vi "main.vi"() -> ()   [LabVIEW 2018]
uses:
  <vilib>/Platform/TimedLoop/XDataNode/timing_clust.ctl
  <vilib>/Platform/TimedLoop/XDataNode/nitl_modes.ctl
  <vilib>/Platform/TimedLoop/XDataNode/wakeup.ctl
  <vilib>/rvi/Emulation/niFpgaGetClockAttributes.vi
  <vilib>/rvi/Emulation/niFpgaSctlEmulationGetInTimedLoop.vi
  <vilib>/rvi/Emulation/niFpgaEmulationReportErrorSimple.vi
  <vilib>/rvi/Emulation/niFpgaProcessEmulError.vi
  <vilib>/rvi/Emulation/niFpgaCriticalErrorInLSC.vi
  <vilib>/Platform/TimedLoop/XDataNode/XDataNode.xnode
  <vilib>/Platform/TimedLoop/XDataNode/XDNodeRunTimeDep.lvlib
panel:
  out "fxp_T_extra2":i32
  out "fxp_T_extra1":i32
  out "fxp_T_pneum":i32
  out "fxp_T_pod":i32
  out "fxp_T_avb_r":i32
  out "fxp_T_avb_p2":i32
  out "fxp_T_avb_p1":i32
  out "fxp_T_piston7":i32
  out "fxp_T_piston6":i32
  out "fxp_T_piston5":i32
  out "fxp_T_piston4":i32
  out "fxp_T_piston3":i32
  out "fxp_T_piston2":i32
  out "fxp_T_piston1":i32
  out "fxp_T_piston0":i32
  out "fuse_avb_p2":bool
  out "fuse_avb_p1":bool
  out "frg_run_state":bool=TRUE
  in  "frg_run":bool=TRUE
  out "cur_thresh_index":u8
  out "cur_thresh_persistence":u32
  out "cur_thresh_ratio":u32
  out "fxp_cur_thresh_max":i32
  out "fxp_cur_thresh_min":i32
  out "fxp_fusion_distance":i32
  in  "fxp_mc_linear_v":i32
  out "fxp_mc_distance":i32
  out "fxp_imu_distance":i32
  in  "fxp_imu_acc":i32
  in  "reset_tape_status":bool
  out "light_sensor_status":u8
  out "enable_checks_state":bool
  in  "enable_checks":bool
  out "fxp_brake_distance":i32
  out "fxp_tape_distance":i32
  out "fxp_brake_force":i32
  out "fxp_P_lp2":i32
  out "fxp_P_lp1":i32
  out "fxp_P_hp2":i32
  out "fxp_P_hp1":i32
  out "fxp_T_cRIO":i32
  out "fxp_tape_velocity":i32
  out "light_R_count":u8
  out "light_L_count":u8
  out "light_BR_count":u8
  out "light_BL_count":u8
  out "light_FL_count":u8
  in  "hvr_4":bool
  in  "hvr_3":bool
  in  "hvr_2":bool
  in  "hvr_1":bool
  in  "avb_shutoff_res":bool
  in  "avb_shutoff_prim_2":bool
  in  "avb_shutoff_prim_1":bool
  in  "iso_led_2":bool
  in  "iso_led_1":bool
  out "avb_shutoff_r_state":bool
  out "avb_shutoff_p2_state":bool
  out "avb_shutoff_p1_state":bool
  out "iso_led_2_state":bool
  out "iso_led_1_state":bool
  out "HVR_4_state":bool
  out "HVR_3_state":bool
  out "HVR_2_state":bool
  out "HVR_1_state":bool
  out "drain_valve_state":bool
  out "brake_state":bool
  out "fxp_voltage_r":i32
  out "fxp_voltage_p2":i32
  out "fxp_voltage_p1":i32
  out "fault_long_3":u64
  out "fault_long_2":u64
  out "soft_fault":u64
  out "hard_fault":u64
  in  "value":fxp<+/-,32,16>
  in  "thresh_read_index":u8
  in  "thresh_reset":bool
  in  "thresh_reset_index":u8
  in  "thresh_latch_new":bool
  in  "thresh_f_ratio":u32
  in  "thresh_persistence":u32
  in  "fxp_thresh_new_max":i32
  in  "fxp_thresh_new_min":i32
  in  "thresh_write_index":u8
  in  "stop":bool
  out "fxp_current_r":i32
  out "fxp_current_p2":i32
  out "fxp_current_p1":i32
  in  "actuate_drain":bool
  in  "actuate_brakes":bool
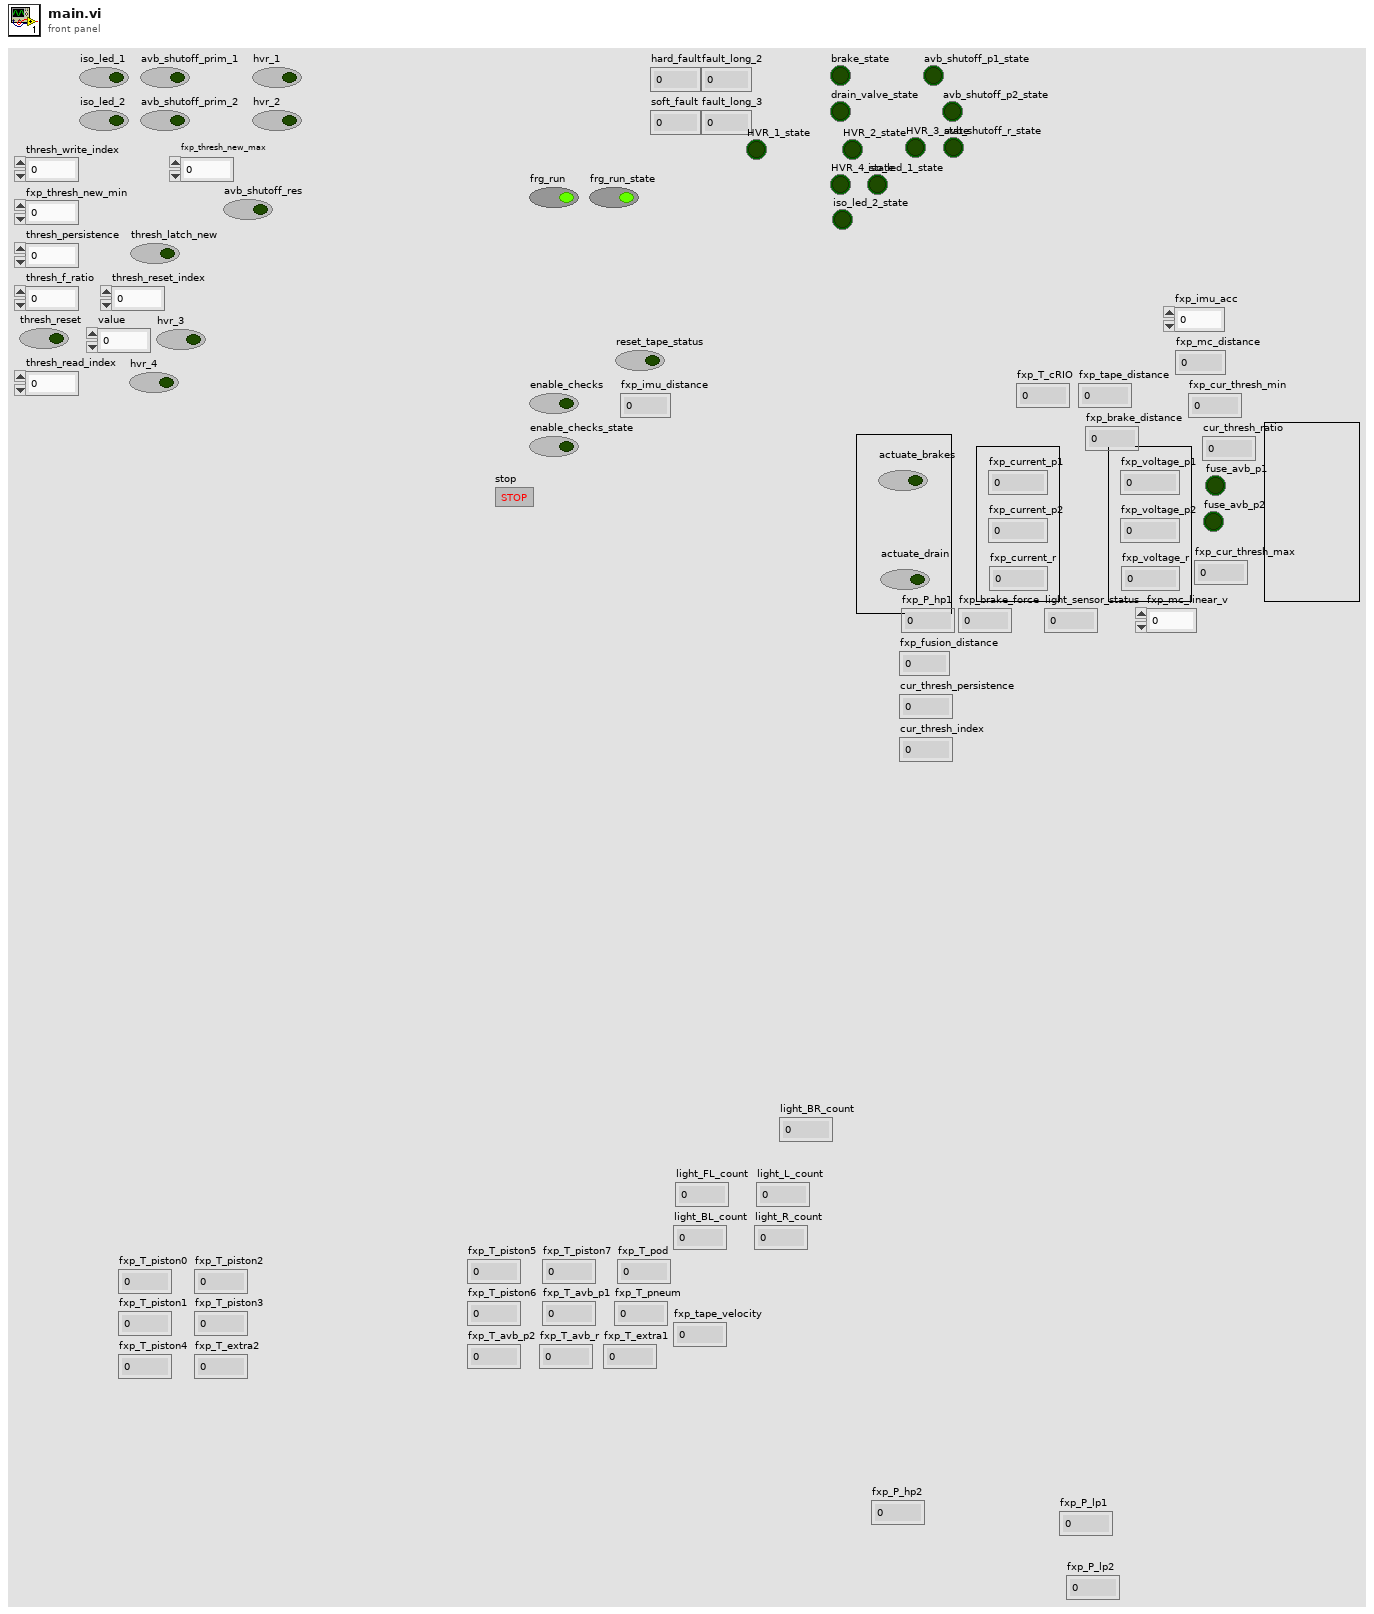
[diagram p1: front panel]
types:
  T1 = typedef "XDNodeRunTimeDep.lvlib/timing_clust.ctl" = cluster{"Expected End [f-1]":u64, "Actual End [f-1]":u64, "Finished Late? [f-1]":bool, "Expected End [i-1]":u64, "Actual End [i-1]":u64, "Finished Late? [i-1]":bool, "Expected Start [i]":u64, "Actual Start [i]":u64, "Expected Start [f]":u64, "Actual Start [f]":u64, "Source Name":string, "Structure Name":string, "Period":i64, "Deadline":i64, "Offset":i64, "Start":i64, "Priority":i32, "Timeout":i32, "Mode":T2, "Wakeup Reason":T3, "Error":errorcluster, "Source Type":string, "Secondary Source Type":string, "Global End Time":u64, "Global Start Time":u64, "Frame Duration":u64, "Iteration Duration":u64, "Assigned CPU":i32, "I/O Scan Engine Mode":u32}
  T2 = typedef "XDNodeRunTimeDep.lvlib/nitl_modes.ctl" = enum32{"No Change", "Process missed periods, maintain original phase", "Discard missed periods, maintain original phase", "Process missed periods, ignore original phase", "Discard missed periods, ignore original phase"}
  T3 = typedef "XDNodeRunTimeDep.lvlib/wakeup.ctl" = enum32{"Normal", "Aborted", "Asynchronous wakeup", "Timing source error", "Timed loop error", "Timeout"}
  T4 = typedef "validated_analog.ctl" = cluster{"valid":bool, "analog":fxp<+/-,24,5>}
  T5 = typedef "validated_bool.ctl" = cluster{"valid":bool, "bool":bool}
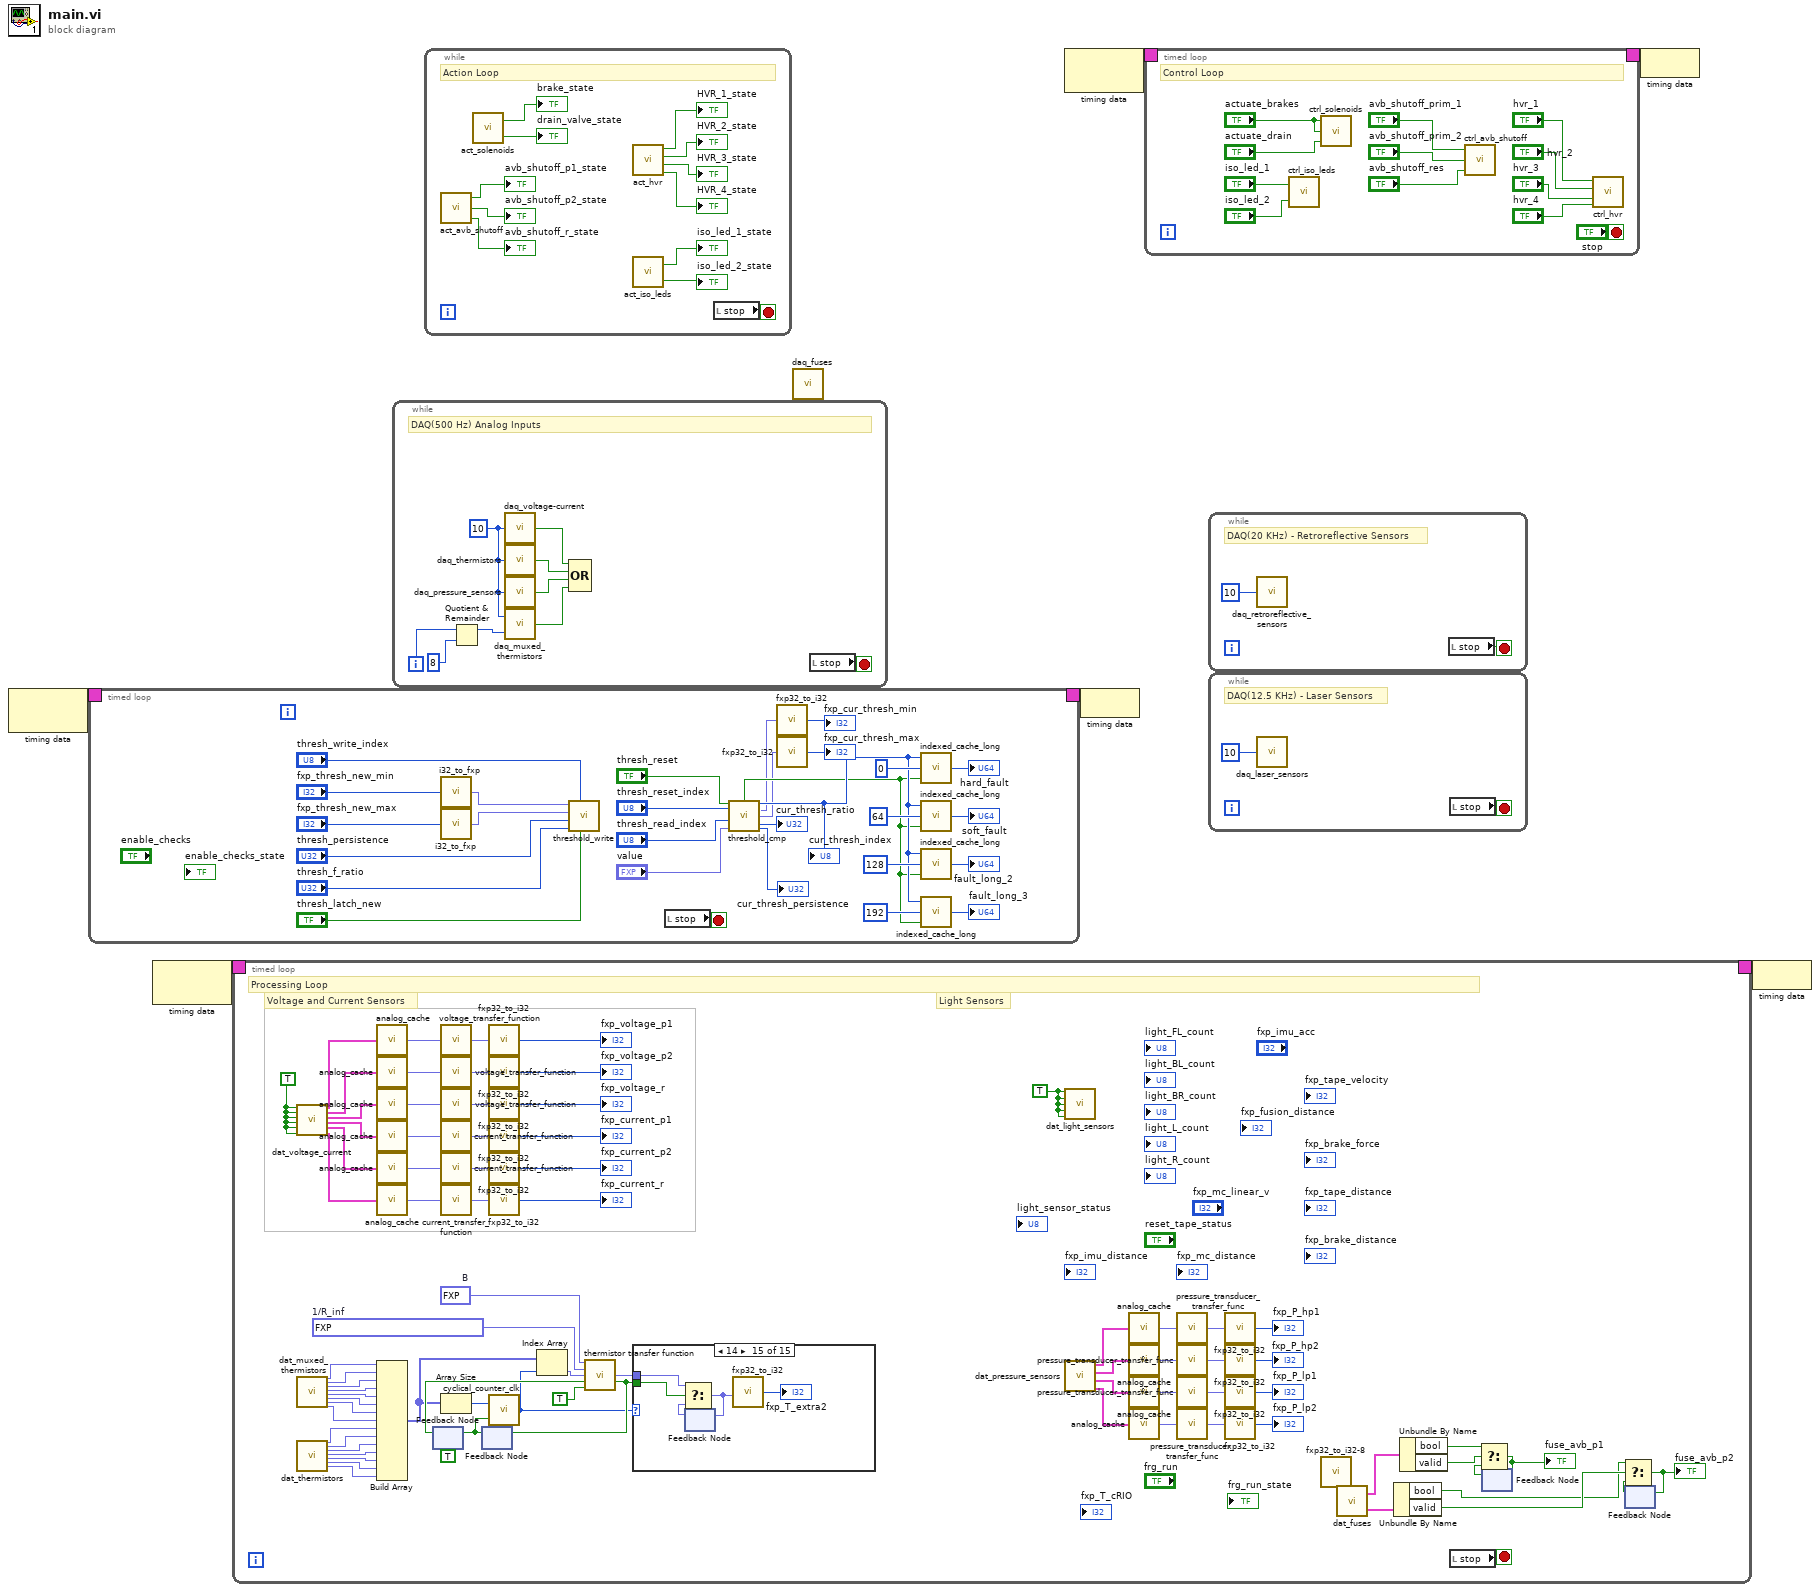
[diagram p0: block diagram]
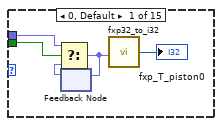
[diagram p2: hidden frame]
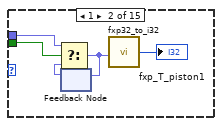
[diagram p3: hidden frame]
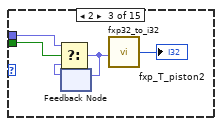
[diagram p4: hidden frame]
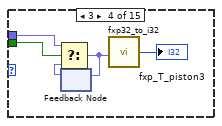
[diagram p5: hidden frame]
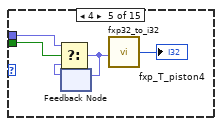
[diagram p6: hidden frame]
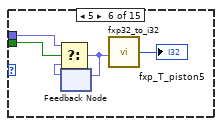
[diagram p7: hidden frame]
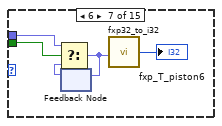
[diagram p8: hidden frame]
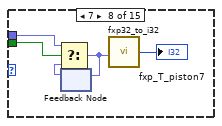
[diagram p9: hidden frame]
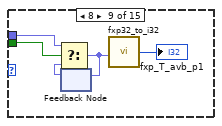
[diagram p10: hidden frame]
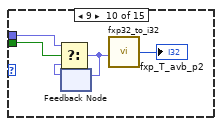
[diagram p11: hidden frame]
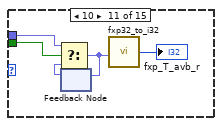
[diagram p12: hidden frame]
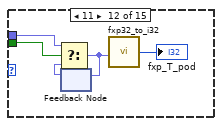
[diagram p13: hidden frame]
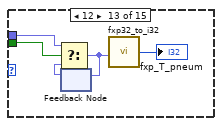
[diagram p14: hidden frame]
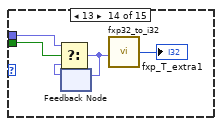
[diagram p15: hidden frame]
diagram:
  n1 = node-c288() -> (w2:T1)  [unwired: 1 in]
  n2 = timed-loop {
    timing: w2 -> [_]
    timing-out: [_] -> w1
    stop <- w35 stop-if-true
    n3 = call "i32_to_fxp.vi"("32bit integer"="fxp_thresh_new_min") -> ("fxp32_16"=w14:fxp<+/-,32,16>)
    n4 = call "i32_to_fxp.vi"("32bit integer"="fxp_thresh_new_max") -> ("fxp32_16"=w13:fxp<+/-,32,16>)
    n5 = call "threshold_write.vi"("thresh_latch"="thresh_latch_new", "thresh_index"="thresh_write_index", "thresh_f_ratio"="thresh_f_ratio", "thresh_persistence"="thresh_persistence", "thresh_new_max"=w13, "thresh_new_min"=w14) -> ()  [unwired: 4 in]
    n6 = local read "stop"() -> (w35:bool)
    n7 = call "threshold_cmp.vi"("thresh_reset"="thresh_reset", "thresh_reset_index"="thresh_reset_index", "index"="thresh_read_index", "value"="value") -> ("thresh_fault"=w21:bool, "current_index"=w22:u8, "current_minimum"=w10:fxp<+/-,32,16>, "current_maximum"=w9:fxp<+/-,32,16>, "current_ratio"=→"cur_thresh_ratio":u32, "current_persistence"=→"cur_thresh_persistence":u32)  [unwired: 6 in]
    "cur_thresh_index" <- w22
    n8 = call "fxp32_to_i32.vi"("fxp32_16"=w10) -> ("32bit integer"=→"fxp_cur_thresh_min":i32)
    n9 = call "fxp32_to_i32.vi"("fxp32_16"=w9) -> ("32bit integer"=→"fxp_cur_thresh_max":i32)
    n10 = call "indexed_cache_long.vi"("bool"=w21, "start index"=u8 0, "index"=w22) -> ("long"=→"hard_fault":u64)  [unwired: 2 in]
    n11 = call "indexed_cache_long.vi"("bool"=w21, "start index"=u8 64, "index"=w22) -> ("long"=→"soft_fault":u64)  [unwired: 2 in]
    n12 = call "indexed_cache_long.vi"("bool"=w21, "start index"=u8 128, "index"=w22) -> ("long"=→"fault_long_2":u64)  [unwired: 2 in]
    n13 = call "indexed_cache_long.vi"("bool"=w21, "start index"=u8 192, "index"=w22) -> ("long"=→"fault_long_3":u64)  [unwired: 2 in]
  }
  n14 = node-c288() -> (w4:T1)  [unwired: 1 in]
  n15 = timed-loop {
    timing: w4 -> [_]
    timing-out: [_] -> w3
    stop <- w111 stop-if-true
    w47 = fxp<+,32,7> 10.047783523797989  # 1/R_inf
    w48 = fxp<+/-,32,16> 3434.0  # B
    w91 = TRUE ("FL-Ready for Output")
    w92 = TRUE
    # "Voltage and Current Sensors"
    # "Light Sensors"
    # "Processing Loop"
    n16 = call "dat_voltage_current.vi"("P1-V Ready for Output"=w92, "P2-V Ready for Output"=w92, "R-V Ready for Output"=w92, "P1-C Ready for Output"=w92, "P2-C Ready for Output"=w92, "R-C Ready for Output"=w92) -> ("P1-V"=w98:T4, "P2-V"=w93:T4, "R-V"=w94:T4, "P1-C"=w95:T4, "P2-C"=w96:T4, "R-C"=w97:T4)  [unwired: 8 in]
    n17 = call "dat_muxed_thermistors.vi"() -> ("v_piston_0"=w64:fxp<+/-,24,5>, "v_piston_1"=w63:fxp<+/-,24,5>, "v_piston_2"=w62:fxp<+/-,24,5>, "v_piston_3"=w61:fxp<+/-,24,5>, "v_piston_4"=w60:fxp<+/-,24,5>, "v_piston_5"=w59:fxp<+/-,24,5>, "v_piston_6"=w58:fxp<+/-,24,5>, "v_piston_7"=w57:fxp<+/-,24,5>)  [unwired: 20 in]
    n18 = call "dat_thermistors.vi"() -> ("v_pb_1_t"=w56:fxp<+/-,24,5>, "v_pb_2_t"=w55:fxp<+/-,24,5>, "v_rb_t"=w54:fxp<+/-,24,5>, "v_pod_t"=w53:fxp<+/-,24,5>, "v_pneum_tank_t"=w52:fxp<+/-,24,5>, "v_extra_1_t"=w51:fxp<+/-,24,5>, "v_extra_2_t"=w50:fxp<+/-,24,5>)  [unwired: 20 in, 1 out]
    n19 = call "analog_cache.vi"("Cluster"=w98) -> ("$_val"=w104:fxp<+/-,24,5>)
    n20 = call "analog_cache.vi"("Cluster"=w93) -> ("$_val"=w103:fxp<+/-,24,5>)
    n21 = call "analog_cache.vi"("Cluster"=w94) -> ("$_val"=w102:fxp<+/-,24,5>)
    n22 = call "analog_cache.vi"("Cluster"=w95) -> ("$_val"=w101:fxp<+/-,24,5>)
    n23 = call "analog_cache.vi"("Cluster"=w96) -> ("$_val"=w100:fxp<+/-,24,5>)
    n24 = call "analog_cache.vi"("Cluster"=w97) -> ("$_val"=w99:fxp<+/-,24,5>)
    n25 = Build Array(w64, w63, w62, w61, w60, w59, w58, w57, w56, w55, w54, w53, w52, w51, w50) -> (w38:fxp<+/-,24,5>[])
    n26 = feedback #1(TRUE ("ready for input")) -> (w42:bool)
    n27 = call "voltage_transfer_function.vi"("V_in"=w104) -> ("V"=w107:fxp<+/-,32,16>)
    n28 = call "voltage_transfer_function.vi"("V_in"=w103) -> ("V"=w106:fxp<+/-,32,16>)
    n29 = call "voltage_transfer_function.vi"("V_in"=w102) -> ("V"=w105:fxp<+/-,32,16>)
    n30 = call "current_transfer_function.vi"("V_in"=w101) -> ("I"=w114:fxp<+/-,32,16>)
    n31 = call "current_transfer_function.vi"("V_in"=w100) -> ("I"=w113:fxp<+/-,32,16>)
    n32 = call "current_transfer_function.vi"("V_in"=w99) -> ("I"=w112:fxp<+/-,32,16>)
    n33 = Array Size(array=w38) -> (size(s)=w45:i32)
    n34 = feedback #2() -> (w40:bool)  [unwired: 1 in]
    n35 = feedback-in #1(w40) -> ()
    n36 = call "fxp32_to_i32.vi"("fxp32_16"=w107) -> ("32bit integer"=→"fxp_voltage_p1":i32)
    n37 = call "fxp32_to_i32.vi"("fxp32_16"=w106) -> ("32bit integer"=→"fxp_voltage_p2":i32)
    n38 = call "fxp32_to_i32.vi"("fxp32_16"=w105) -> ("32bit integer"=→"fxp_voltage_r":i32)
    n39 = call "fxp32_to_i32.vi"("fxp32_16"=w114) -> ("32bit integer"=→"fxp_current_p1":i32)
    n40 = call "fxp32_to_i32.vi"("fxp32_16"=w113) -> ("32bit integer"=→"fxp_current_p2":i32)
    n41 = call "fxp32_to_i32.vi"("fxp32_16"=w112) -> ("32bit integer"=→"fxp_current_r":i32)
    n42 = call "cyclical_counter_clk.vi"("clk"=w40, "Mod"=w45) -> ("Count"=w39:u16)
    n43 = Index Array(array=w38, index=w39) -> (element=w49:fxp<+/-,24,5>)
    n44 = call "thermistor transfer function.vi"("B"=w48, "1/R_inf"=w47, "V"=w49, "input valid"=w42, "ready for output (T)"=TRUE) -> ("Temperature"=w46:fxp<+/-,32,16>, "output valid"=w41:bool)  [unwired: 8 in, 1 out]
    n45 = feedback-in #2(w41) -> ()
    n46 = case shown="14" w39 {
      tunnel: w41 -> [w119 w124 w129 w134 w139 w144 w149 w154 w159 w164 w169 w174 w179 w184 w189]
      tunnel: w46 -> [w122 w127 w132 w137 w142 w147 w152 w157 w162 w167 w172 w177 w182 w187 w192]
      frame 0, Default {
        n47 = feedback #3() -> (w120:fxp<+/-,32,16>)  [unwired: 1 in]
        n48 = Select(t=w122, s=w119, f=w120) -> (s? t:f=w121:fxp<+/-,32,16>)
        n49 = feedback-in #3(w121) -> ()
        n50 = call "fxp32_to_i32.vi"("fxp32_16"=w121) -> ("32bit integer"=→"fxp_T_piston0":i32)
      }
      frame 1 {
        n51 = feedback #4() -> (w125:fxp<+/-,32,16>)  [unwired: 1 in]
        n52 = Select(t=w127, s=w124, f=w125) -> (s? t:f=w126:fxp<+/-,32,16>)
        n53 = feedback-in #4(w126) -> ()
        n54 = call "fxp32_to_i32.vi"("fxp32_16"=w126) -> ("32bit integer"=→"fxp_T_piston1":i32)
      }
      frame 2 {
        n55 = feedback #5() -> (w130:fxp<+/-,32,16>)  [unwired: 1 in]
        n56 = Select(t=w132, s=w129, f=w130) -> (s? t:f=w131:fxp<+/-,32,16>)
        n57 = feedback-in #5(w131) -> ()
        n58 = call "fxp32_to_i32.vi"("fxp32_16"=w131) -> ("32bit integer"=→"fxp_T_piston2":i32)
      }
      frame 3 {
        n59 = feedback #6() -> (w135:fxp<+/-,32,16>)  [unwired: 1 in]
        n60 = Select(t=w137, s=w134, f=w135) -> (s? t:f=w136:fxp<+/-,32,16>)
        n61 = feedback-in #6(w136) -> ()
        n62 = call "fxp32_to_i32.vi"("fxp32_16"=w136) -> ("32bit integer"=→"fxp_T_piston3":i32)
      }
      frame 4 {
        n63 = feedback #7() -> (w140:fxp<+/-,32,16>)  [unwired: 1 in]
        n64 = Select(t=w142, s=w139, f=w140) -> (s? t:f=w141:fxp<+/-,32,16>)
        n65 = feedback-in #7(w141) -> ()
        n66 = call "fxp32_to_i32.vi"("fxp32_16"=w141) -> ("32bit integer"=→"fxp_T_piston4":i32)
      }
      frame 5 {
        n67 = feedback #8() -> (w145:fxp<+/-,32,16>)  [unwired: 1 in]
        n68 = Select(t=w147, s=w144, f=w145) -> (s? t:f=w146:fxp<+/-,32,16>)
        n69 = feedback-in #8(w146) -> ()
        n70 = call "fxp32_to_i32.vi"("fxp32_16"=w146) -> ("32bit integer"=→"fxp_T_piston5":i32)
      }
      frame 6 {
        n71 = feedback #9() -> (w150:fxp<+/-,32,16>)  [unwired: 1 in]
        n72 = Select(t=w152, s=w149, f=w150) -> (s? t:f=w151:fxp<+/-,32,16>)
        n73 = feedback-in #9(w151) -> ()
        n74 = call "fxp32_to_i32.vi"("fxp32_16"=w151) -> ("32bit integer"=→"fxp_T_piston6":i32)
      }
      frame 7 {
        n75 = feedback #10() -> (w155:fxp<+/-,32,16>)  [unwired: 1 in]
        n76 = Select(t=w157, s=w154, f=w155) -> (s? t:f=w156:fxp<+/-,32,16>)
        n77 = feedback-in #10(w156) -> ()
        n78 = call "fxp32_to_i32.vi"("fxp32_16"=w156) -> ("32bit integer"=→"fxp_T_piston7":i32)
      }
      frame 8 {
        n79 = feedback #11() -> (w160:fxp<+/-,32,16>)  [unwired: 1 in]
        n80 = Select(t=w162, s=w159, f=w160) -> (s? t:f=w161:fxp<+/-,32,16>)
        n81 = feedback-in #11(w161) -> ()
        n82 = call "fxp32_to_i32.vi"("fxp32_16"=w161) -> ("32bit integer"=→"fxp_T_avb_p1":i32)
      }
      frame 9 {
        n83 = feedback #12() -> (w165:fxp<+/-,32,16>)  [unwired: 1 in]
        n84 = Select(t=w167, s=w164, f=w165) -> (s? t:f=w166:fxp<+/-,32,16>)
        n85 = feedback-in #12(w166) -> ()
        n86 = call "fxp32_to_i32.vi"("fxp32_16"=w166) -> ("32bit integer"=→"fxp_T_avb_p2":i32)
      }
      frame 10 {
        n87 = feedback #13() -> (w170:fxp<+/-,32,16>)  [unwired: 1 in]
        n88 = Select(t=w172, s=w169, f=w170) -> (s? t:f=w171:fxp<+/-,32,16>)
        n89 = feedback-in #13(w171) -> ()
        n90 = call "fxp32_to_i32.vi"("fxp32_16"=w171) -> ("32bit integer"=→"fxp_T_avb_r":i32)
      }
      frame 11 {
        n91 = feedback #14() -> (w175:fxp<+/-,32,16>)  [unwired: 1 in]
        n92 = Select(t=w177, s=w174, f=w175) -> (s? t:f=w176:fxp<+/-,32,16>)
        n93 = feedback-in #14(w176) -> ()
        n94 = call "fxp32_to_i32.vi"("fxp32_16"=w176) -> ("32bit integer"=→"fxp_T_pod":i32)
      }
      frame 12 {
        n95 = feedback #15() -> (w180:fxp<+/-,32,16>)  [unwired: 1 in]
        n96 = Select(t=w182, s=w179, f=w180) -> (s? t:f=w181:fxp<+/-,32,16>)
        n97 = feedback-in #15(w181) -> ()
        n98 = call "fxp32_to_i32.vi"("fxp32_16"=w181) -> ("32bit integer"=→"fxp_T_pneum":i32)
      }
      frame 13 {
        n99 = feedback #16() -> (w185:fxp<+/-,32,16>)  [unwired: 1 in]
        n100 = Select(t=w187, s=w184, f=w185) -> (s? t:f=w186:fxp<+/-,32,16>)
        n101 = feedback-in #16(w186) -> ()
        n102 = call "fxp32_to_i32.vi"("fxp32_16"=w186) -> ("32bit integer"=→"fxp_T_extra1":i32)
      }
      frame 14 {
        n103 = feedback #17() -> (w190:fxp<+/-,32,16>)  [unwired: 1 in]
        n104 = Select(t=w192, s=w189, f=w190) -> (s? t:f=w191:fxp<+/-,32,16>)
        n105 = feedback-in #17(w191) -> ()
        n106 = call "fxp32_to_i32.vi"("fxp32_16"=w191) -> ("32bit integer"=→"fxp_T_extra2":i32)
      }
    }
    n107 = call "dat_light_sensors.vi"("FL-Ready for Output"=w91, "BL-Ready for Output 2"=w91, "BR-Ready for Output 3"=w91, "L-Ready for Output 4"=w91, "R-Ready for Output 5"=w91) -> ()  [unwired: 6 in, 5 out]
    n108 = call "dat_pressure_sensors.vi"() -> ("P_LP_2"=w77:T4, "P_LP_1"=w75:T4, "P_HP_2"=w76:T4, "P_HP_1"=w90:T4)  [unwired: 8 in]
    n109 = call "analog_cache.vi"("Cluster"=w90) -> ("$_val"=w89:fxp<+/-,24,5>)
    n110 = call "analog_cache.vi"("Cluster"=w76) -> ("$_val"=w86:fxp<+/-,24,5>)
    n111 = call "analog_cache.vi"("Cluster"=w75) -> ("$_val"=w83:fxp<+/-,24,5>)
    n112 = call "analog_cache.vi"("Cluster"=w77) -> ("$_val"=w80:fxp<+/-,24,5>)
    n113 = call "pressure_transducer_transfer_func.vi"("p_v"=w89) -> ("pressure"=w88:fxp<+/-,32,16>)
    n114 = call "pressure_transducer_transfer_func.vi"("p_v"=w86) -> ("pressure"=w85:fxp<+/-,32,16>)
    n115 = call "pressure_transducer_transfer_func.vi"("p_v"=w83) -> ("pressure"=w82:fxp<+/-,32,16>)
    n116 = call "pressure_transducer_transfer_func.vi"("p_v"=w80) -> ("pressure"=w79:fxp<+/-,32,16>)
    n117 = call "fxp32_to_i32.vi"("fxp32_16"=w88) -> ("32bit integer"=→"fxp_P_hp1":i32)
    n118 = call "fxp32_to_i32.vi"("fxp32_16"=w85) -> ("32bit integer"=→"fxp_P_hp2":i32)
    n119 = call "fxp32_to_i32.vi"("fxp32_16"=w82) -> ("32bit integer"=→"fxp_P_lp1":i32)
    n120 = call "fxp32_to_i32.vi"("fxp32_16"=w79) -> ("32bit integer"=→"fxp_P_lp2":i32)
    n121 = call "fxp32_to_i32-8.vi"() -> ()  [unwired: 20 in, 8 out]
    n122 = call "dat_fuses.vi"() -> ("fuse_av_2"=w73:T5, "fuse_av_1"=w74:T5)  [unwired: 2 in]
    n123 = Unbundle By Name(w73) -> ("bool"=w65:bool, "valid"=w72:bool)
    n124 = Unbundle By Name(w74) -> ("bool"=w70:bool, "valid"=w71:bool)
    n125 = local read "stop"() -> (w111:bool)
    n126 = feedback #18() -> (w68:bool)  [unwired: 1 in]
    n127 = Select(t=w70, s=w71, f=w68) -> (s? t:f=w69:bool)
    "fuse_avb_p1" <- w69
    n128 = feedback-in #18(w69) -> ()
    n129 = feedback #19() -> (w66:bool)  [unwired: 1 in]
    n130 = Select(t=w65, s=w72, f=w66) -> (s? t:f=w67:bool)
    "fuse_avb_p2" <- w67
    n131 = feedback-in #19(w67) -> ()
  }
  n132 = while {
    i -> [w203]
    stop <- w195 stop-if-true
    w200 = 10 ("Timeout")
    # "DAQ(500 Hz) Analog Inputs"
    n133 = Quotient & Remainder(x=w203, y=8) -> (x-y*floor(x/y)=w201:i32)  [unwired: 1 out]
    n134 = call "daq_voltage-current.vi"("Timeout"=w200) -> ("FIFO_timeout"=w199:bool)
    n135 = call "daq_thermistors.vi"("Timeout"=w200) -> ("FIFO_timeout"=w196:bool)
    n136 = call "daq_pressure_sensors.vi"("Timeout"=w200) -> ("FIFO_timeout"=w197:bool)
    n137 = call "daq_muxed_thermistors.vi"("index"=w201, "Timeout"=w200) -> ("Timed Out?"=w198:bool)
    n138 = Compound Arithmetic op=OR(w199, w196, w197, w198) -> ()  [unwired: 1 out]
    n139 = local read "stop"() -> (w195:bool)
  }
  n140 = while {
    stop <- w204 stop-if-true
    # "Action Loop"
    n141 = call "act_avb_shutoff.vi"() -> ("avb_shutoff_r"=→"avb_shutoff_r_state":bool, "avb_shutoff_p2"=→"avb_shutoff_p2_state":bool, "avb_shutoff_p1"=→"avb_shutoff_p1_state":bool)
    n142 = call "act_solenoids.vi"() -> ("drain_valve_state"=→"drain_valve_state":bool, "brake_state"=→"brake_state":bool)  [unwired: 2 in]
    n143 = call "act_hvr.vi"() -> ("HVR_4"=→"HVR_4_state":bool, "HVR_3"=→"HVR_3_state":bool, "HVR_2"=→"HVR_2_state":bool, "HVR_1"=→"HVR_1_state":bool)  [unwired: 8 in]
    n144 = call "act_iso_leds.vi"() -> ("iso_led_2"=→"iso_led_2_state":bool, "iso_led_1"=→"iso_led_1_state":bool)  [unwired: 2 in]
    n145 = local read "stop"() -> (w204:bool)
  }
  n146 = call "daq_fuses.vi"() -> ()  [unwired: 1 in, 1 out]
  n147 = node-c288() -> (w6:T1)  [unwired: 1 in]
  n148 = node-c288(w1) -> ()
  n149 = timed-loop {
    timing: w6 -> [_]
    timing-out: [_] -> w5
    stop <- "stop" stop-if-true
    # "Control Loop"
    n150 = call "ctrl_iso_leds.vi"("iso_led_2"="iso_led_2", "iso_led_1"="iso_led_1") -> ()  [unwired: 1 in]
    n151 = call "ctrl_solenoids.vi"("drain"="actuate_drain", "brake_2"="actuate_brakes", "brake_1"="actuate_brakes") -> ()
    n152 = call "ctrl_avb_shutoff.vi"("avb_shutoff_res"="avb_shutoff_res", "avb_shutoff_prim_2"="avb_shutoff_prim_2", "avb_shutoff_prim_1"="avb_shutoff_prim_1") -> ()
    n153 = call "ctrl_hvr.vi"("hvr_4"="hvr_4", "hvr_3"="hvr_3", "hvr_2"="hvr_2", "hvr_1"="hvr_1") -> ()  [unwired: 8 in]
  }
  n154 = while {
    stop <- w230 stop-if-true
    # "DAQ(20 KHz) - Retroreflective Sensors"
    n155 = call "daq_retroreflective_sensors.vi"("Timeout"=10) -> ()  [unwired: 1 out]
    n156 = local read "stop"() -> (w230:bool)
  }
  n157 = while {
    stop <- w232 stop-if-true
    # "DAQ(12.5 KHz) - Laser Sensors"
    n158 = call "daq_laser_sensors.vi"("Timeout"=10) -> ()  [unwired: 1 out]
    n159 = local read "stop"() -> (w232:bool)
  }
  n160 = node-c288(w5) -> ()
  n161 = node-c288(w3) -> ()
